vi "getLevel.vi"(8 "error in (no error)":errorcluster, 11 "Tank in":refnum<class "Tank.lvclass">) -> (0 "error out":errorcluster, 2 "Level":dbl, 3 "Tank out":refnum<class "Tank.lvclass">)   [LabVIEW 2018, in "Tank.lvclass"]
uses:
  Tank.lvclass
  Tank.lvclass/Tank.ctl
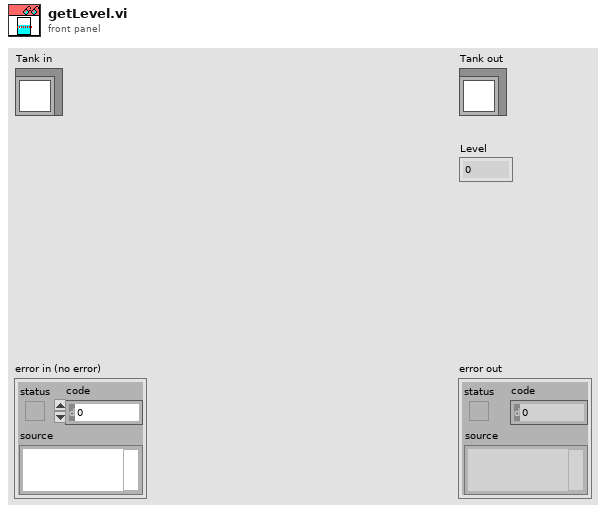
[diagram p1: front panel]
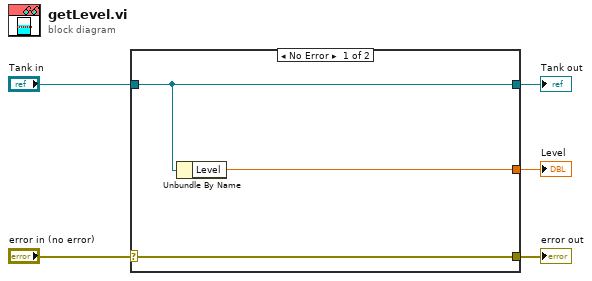
[diagram p0: block diagram]
diagram:
  n1 = case shown="No Error" "error in (no error)" {
    selector: "error in (no error)" -> [w8 w9]
    tunnel: [w8 w9] -> w4
    tunnel: [w7 w10] -> w2
    tunnel: "Tank in" -> [w7 w10]
    tunnel: [w6 _] -> w1
    frame No Error {
      n2 = Unbundle By Name(w7) -> ("Level"=w6:dbl)
    }
    frame Error {
    }
  }
  "error out" <- w4
  "Tank out" <- w2
  "Level" <- w1
